vi "Do.vi"(8 "error in (no error)":errorcluster, 10 "Actor in":refnum<class "Actor.lvclass">, 11 "Change DC":refnum<class "Change DC MSG.lvclass">) -> (0 "error out":errorcluster, 2 "Actor out":refnum<class "Actor.lvclass">)   [LabVIEW 2014, in "eCRDS Library.lvlib" / "Change DC MSG.lvclass"]
doc: "(<B>Filename</B>: Actor Framework.lvlib:Message.lvclass:Do.vi)\n\nDefines what a message does when it is received by an actor. Generally, a message instructs an actor to invoke one of its methods. By default, this method does nothing. A child class must override it to define behavior. Create a child class by using the Actor Framework Message Maker dialog box."
uses:
  Change DC MSG.lvclass
  <vilib>/ActorFramework/Actor/Actor.lvclass
  Change DC MSG.lvclass/Change DC MSG.ctl
  Instr Actor/Instr Actor.lvclass
  Commands/Update Blue DC/Update Blue DC.lvclass
  Commands/Update Blue DC/Update Blue DC.lvclass/Update Blue DC.ctl
  Commands/Update Red DC/Update Red DC.lvclass
  Commands/Update Red DC/Update Red DC.lvclass/Update Red DC.ctl
  SuperActor/SuperActor.lvclass/SuperActor.ctl
  SuperActor/Read CVT Session.vi
  SuperActor/Read Log Session.vi
  <userlib>/_Session Fwk/Session - Root.lvclass
  reusable/Command/Command.lvclass
  reusable/Session APIs/CVT/CVT.lvclass
  reusable/Session APIs/Session Log/System Log.lvclass
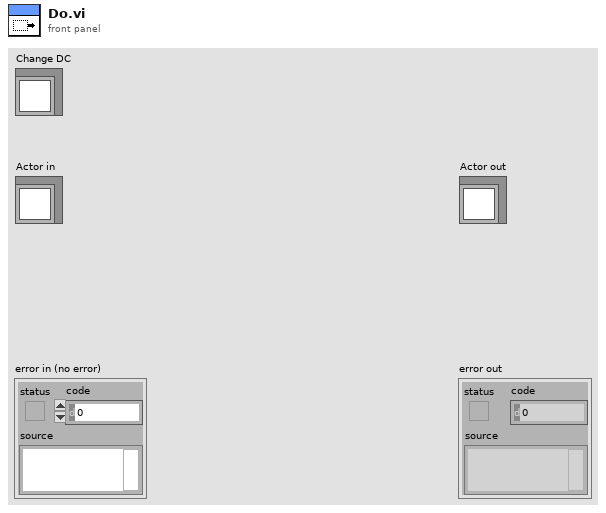
[diagram p1: front panel]
types:
  T1 = typedef "Session - Root.lvclass/Session Handle.ctl" = refnum<data-value>
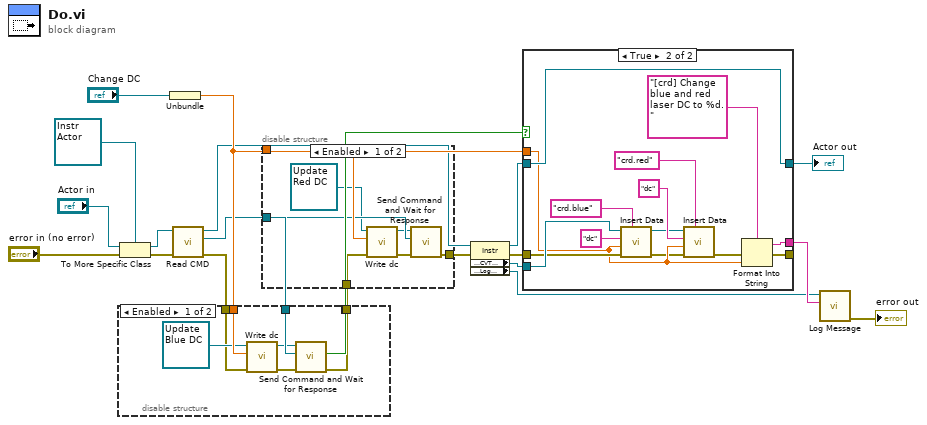
[diagram p0: block diagram]
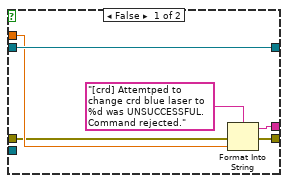
[diagram p4: hidden frame]
diagram:
  n1 = To More Specific Class(target class=refnum<class "Instr Actor.lvclass"> refnum ("Instrument Lib:Instr"), reference="Actor in", error in="error in (no error)") -> (specific class reference=w8:refnum<class "Instr Actor.lvclass">, error out=w7:errorcluster)
  n2 = Unbundle("Change DC") -> (w10:dbl)
  n3 = call "Read CMD.vi"("error in (no error)"=w7, "Instr Actor in"=w8) -> ("error out"=w2:errorcluster, "CMD"=w5:refnum<queue>, "Instr Actor out"=w6:refnum<class "Instr Actor.lvclass">)  [unwired: 7 in]
  n4 = disable-structure shown="Enabled" {
    disable-tunnel: [w28 _] -> w16
    disable-tunnel: w10 -> [w27 _]
    disable-tunnel: w5 -> [w26 _]
    disable-tunnel: [w23 _] -> w3
    disable-tunnel: w2 -> [w22 _]
    frame Enabled {
      n5 = call "Write dc.vi"("error in (no error)"=w22, "dc"=w27, "Update Blue DC in"=refnum<class "Update Blue DC.lvclass"> refnum ("eCRDS Library.lvlib:Update Blue DC.lvclass")) -> ("error out"=w21:errorcluster, "Update Blue DC out"=w25:refnum<class "Update Blue DC.lvclass">)  [unwired: 7 in]
      n6 = call "Send Command and Wait for Response.vi"("error in"=w21, "cmd queue"=w26, "CMD in"=w25) -> ("error out"=w23:errorcluster, "cmd good?"=w28:bool)  [unwired: 6 in, 1 out]
    }
    frame Disabled {
    }
  }
  n7 = disable-structure shown="Enabled" {
    disable-tunnel: w10 -> [w35 _]
    disable-tunnel: w5 -> [w34 _]
    disable-tunnel: [w33 w36] -> w4
    disable-tunnel: w3 -> [w32 w36]
    frame Enabled {
      n8 = call "Write dc.vi"("error in (no error)"=w32, "dc"=w35, "Update Blue DC in"=refnum<class "Update Red DC.lvclass"> refnum ("eCRDS Library.lvlib: Update Red DC.lvclass")) -> ("error out"=w30:errorcluster, "Update Blue DC out"=w31:refnum<class "Update Red DC.lvclass">)  [unwired: 7 in]
      n9 = call "Send Command and Wait for Response.vi"("error in"=w30, "cmd queue"=w34, "CMD in"=w31) -> ("error out"=w33:errorcluster)  [unwired: 6 in, 2 out]
    }
    frame Disabled {
    }
  }
  n10 = property class="Instr"(reference=w6, error in=w4) -> (reference out=w15:refnum<class "Instr Actor.lvclass">, error out=w14:errorcluster, "Accessors:CVT Session"=w11:T1, "Accessors:Log Session"=w12:T1)
  n11 = case shown="True" w16 {
    tunnel: w10 -> [w41 w45]
    tunnel: w15 -> [w42 w56]
    tunnel: [w42 w56] -> w18
    tunnel: w14 -> [w39 w49]
    tunnel: [w38 w53] -> _
    tunnel: [w37 w54] -> w13
    tunnel: w11 -> [_ w51]
    frame False {
      n12 = Format Into String(format string="[crd] Attemtped to change crd blue laser to %d was UNSUCCESSFUL.  Command rejected.", error in=w39, w41) -> (resulting string=w37:string, error out=w38:errorcluster)  [unwired: 1 in]
    }
    frame True {
      n13 = call "Insert Data.vi"("Group"="crd.blue", "error in"=w49, "Data"=w45, "tag"="dc", "CVT Session In"=w51) -> ("error out"=w44:errorcluster, "CVT Session Out"=w46:T1)  [unwired: 5 in]
      n14 = call "Insert Data.vi"("Group"="crd.red", "error in"=w44, "Data"=w45, "tag"="dc", "CVT Session In"=w46) -> ("error out"=w43:errorcluster)  [unwired: 5 in, 1 out]
      n15 = Format Into String(format string="[crd] Change blue and red laser DC to %d.", error in=w43, w45) -> (resulting string=w54:string, error out=w53:errorcluster)  [unwired: 1 in]
    }
  }
  "Actor out" <- w18
  n16 = call "Log Message.vi"("MSG In"=w13, "session in"=w12) -> ("error out"=→"error out":errorcluster)  [unwired: 8 in, 1 out]
